vi "SetClassProperties.vi"(8 "error in (no error)":errorcluster, 11 "Gviewer in":refnum<class "Gviewer.lvclass">) -> (0 "error out":errorcluster, 3 "Gviewer out":refnum<class "Gviewer.lvclass">)   [LabVIEW 2020, in "Sgraph_lib_V1.lvlib" / "Gviewer.lvclass"]
doc: "Update the Graph Properties"
uses:
  Gviewer.lvclass
  Gviewer.lvclass/Gviewer.ctl
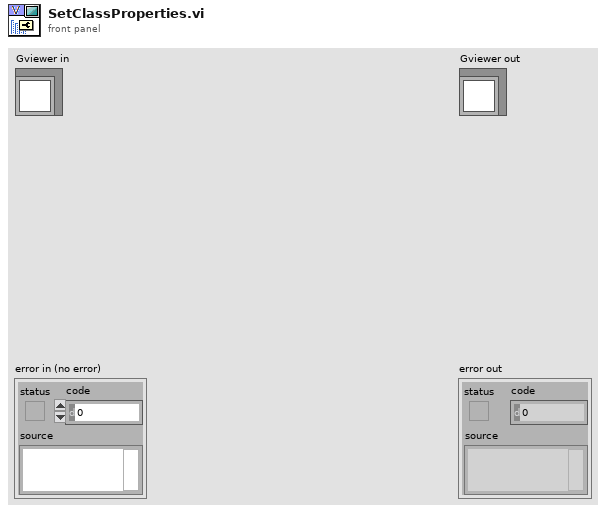
[diagram p1: front panel]
types:
  T1 = typedef "Sgraph_lib_V1.lvlib/Gviewer.lvclass/Typedef_SelProperties.ctl" = cluster{"Color":u32, "LineType":T2, "max":dbl, "min":dbl}
  T2 = typedef "Sgraph_lib_V1.lvlib/Gviewer.lvclass/Typedef_LineType.ctl" = enum16{"num_bare", "num_MinMax_Area", "num_MinMax_Lines", "num_MinMax_Forfor", "num_Max_Area", "num_Max_Line", "num_Max_Forfor", "num_Min_Area", "num_Min_Line", "num_Min_Fosfor", "Boolean_Line_01", "Boolean_Area_01", "Boolean_Fosfor_01", "Boolean_Line_TF", "Boolean_Area_TF", "Boolean_Fosfor_TF", "Boolean_OnOff_Line", "Boolean_OnOff_Area", "Boolean_OnOff_Fosfor", "Boolean_spare", "StringEvent_Line", "StringEvent_TimeLine"}
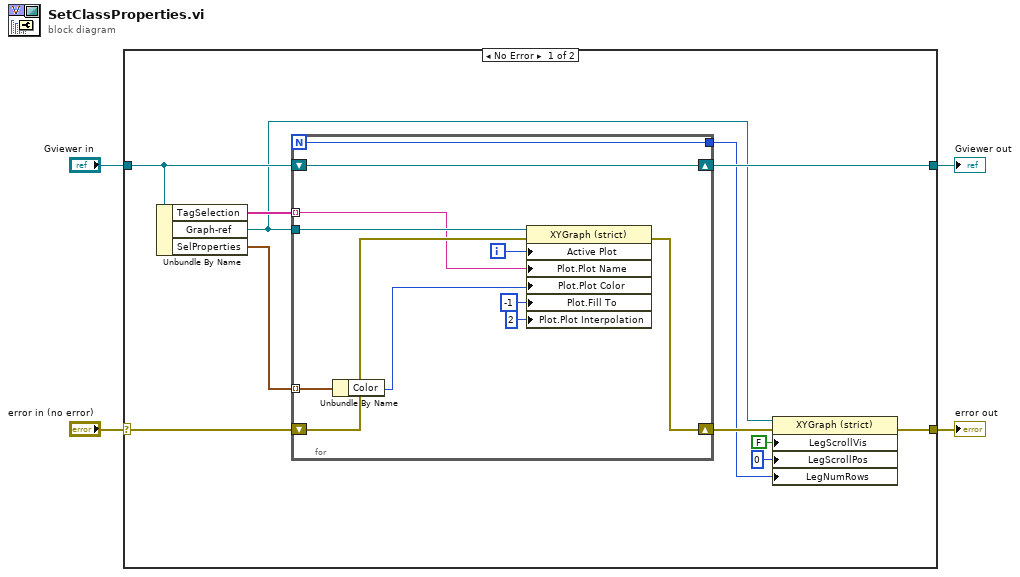
[diagram p0: block diagram]
diagram:
  n1 = case shown="No Error" "error in (no error)" {
    selector: "error in (no error)" -> [w15 w28]
    tunnel: [w6 w28] -> w3
    tunnel: [w11 w27] -> w1
    tunnel: "Gviewer in" -> [w14 w27]
    frame No Error {
      n2 = Unbundle By Name(w14) -> ("TagSelection"=w12:string[], "Graph-ref"=w5:refnum<vi>, "SelProperties"=w13:T1[])
      n3 = for {
        N -> [w22]
        shift-right: [w17] -> w9
        shift-left: w15 -> [w23]
        shift-right: [w25] -> w11
        shift-left: w14 -> [w25]
        tunnel: w13 -> [w26] mode=indexing
        tunnel: w5 -> [w24]
        tunnel: w12 -> [w19] mode=indexing
        tunnel: [w22] -> w7
        i -> [w20]
        n4 = Unbundle By Name(w26) -> ("Color"=w18:u32)
        n5 = property class="XYGraph (strict)"(reference=w24, error in=w23, "Active Plot"=w20, "Plot.Plot Name"=w19, "Plot.Plot Color"=w18, "Plot.Fill To"=i16 -1, "Plot.Plot Interpolation"=u8 2) -> (error out=w17:errorcluster)  [unwired: 1 out]
      }
      n6 = property class="XYGraph (strict)"(reference=w5, error in=w9, "LegScrollVis"=FALSE ("Legend:Scrollbar Visible"), "LegScrollPos"=u32 0 ("Legend:Scroll Position"), "LegNumRows"=w7) -> (error out=w6:errorcluster)  [unwired: 1 out]
    }
    frame Error {
    }
  }
  "error out" <- w3
  "Gviewer out" <- w1
